vi "Test_PXI_Trig2.vi"() -> ()   [LabVIEW 2018]
uses:
  <vilib>/Platform/TimedLoop/XDataNode/timing_clust.ctl
  <vilib>/Platform/TimedLoop/XDataNode/nitl_modes.ctl
  <vilib>/Platform/TimedLoop/XDataNode/wakeup.ctl
  <vilib>/rvi/Emulation/niFpgaGetClockAttributes.vi
  <vilib>/rvi/Emulation/niFpgaSctlEmulationGetInTimedLoop.vi
  <vilib>/rvi/Emulation/niFpgaEmulationReportErrorSimple.vi
  <vilib>/rvi/eio/common/nirviEmuTemplateMethod_errors.vi
  <vilib>/rvi/Emulation/niFpgaCriticalErrorInLSC.vi
  <vilib>/eio/EIONode/EIONode.xnode
  <vilib>/Platform/TimedLoop/XDataNode/XDataNode.xnode
  <vilib>/Platform/TimedLoop/XDataNode/XDNodeRunTimeDep.lvlib
panel:
  out "PXI_Trig0 read":bool
  in  "PXI_Trig0  write":bool
  in  "Sample Clock Commit":bool
  in  "Sample Clock Select":u8
  out "SPI Idle":bool
  out "Configuration Error":bool
  out "Synthesizer Locked":bool
  out "Configured?":bool
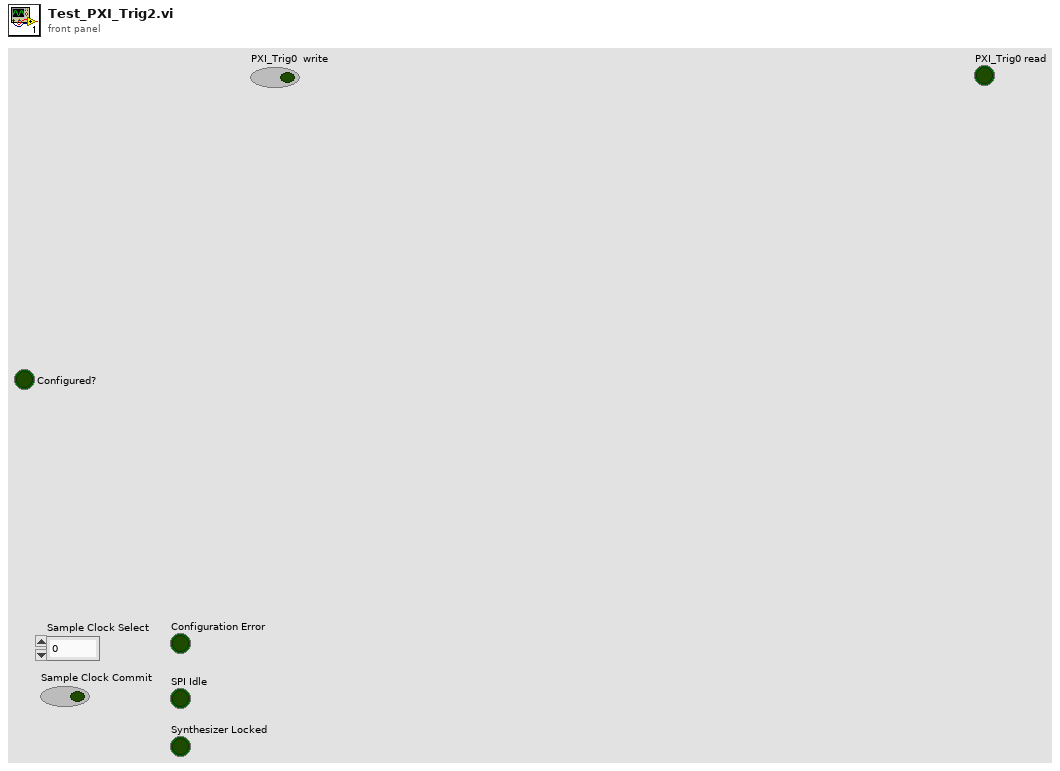
[diagram p1: front panel]
types:
  T1 = typedef "XDNodeRunTimeDep.lvlib/timing_clust.ctl" = cluster{"Expected End [f-1]":u64, "Actual End [f-1]":u64, "Finished Late? [f-1]":bool, "Expected End [i-1]":u64, "Actual End [i-1]":u64, "Finished Late? [i-1]":bool, "Expected Start [i]":u64, "Actual Start [i]":u64, "Expected Start [f]":u64, "Actual Start [f]":u64, "Source Name":string, "Structure Name":string, "Period":i64, "Deadline":i64, "Offset":i64, "Start":i64, "Priority":i32, "Timeout":i32, "Mode":T2, "Wakeup Reason":T3, "Error":errorcluster, "Source Type":string, "Secondary Source Type":string, "Global End Time":u64, "Global Start Time":u64, "Frame Duration":u64, "Iteration Duration":u64, "Assigned CPU":i32, "I/O Scan Engine Mode":u32}
  T2 = typedef "XDNodeRunTimeDep.lvlib/nitl_modes.ctl" = enum32{"No Change", "Process missed periods, maintain original phase", "Discard missed periods, maintain original phase", "Process missed periods, ignore original phase", "Discard missed periods, ignore original phase"}
  T3 = typedef "XDNodeRunTimeDep.lvlib/wakeup.ctl" = enum32{"Normal", "Aborted", "Asynchronous wakeup", "Timing source error", "Timed loop error", "Timeout"}
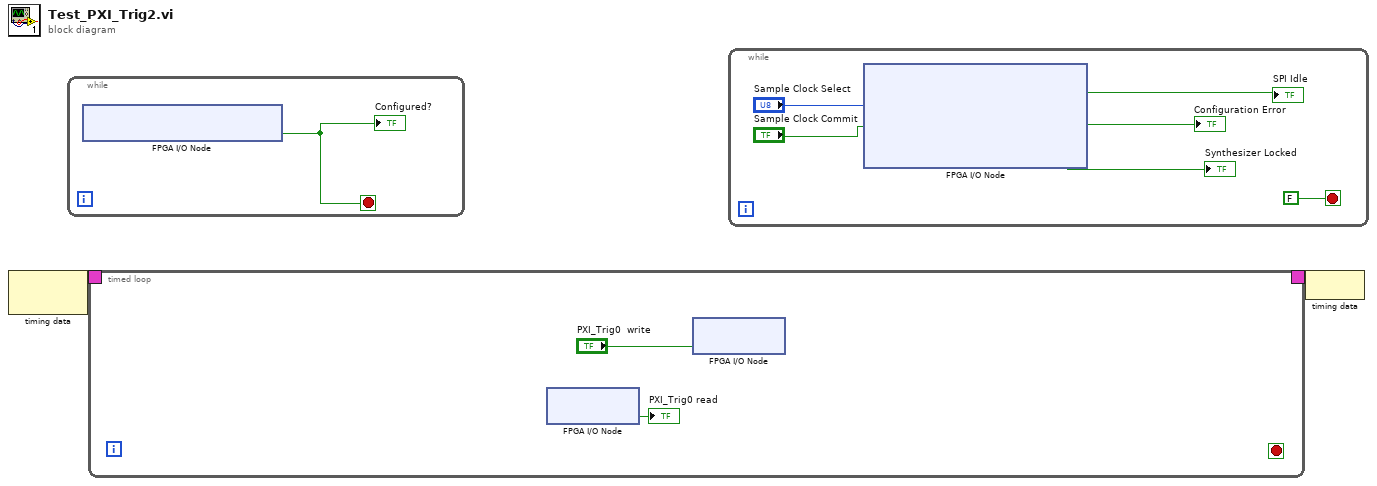
[diagram p0: block diagram]
diagram:
  n1 = node-c288() -> (w2:T1)  [unwired: 1 in]
  n2 = while {
    stop <- w3 stop-if-true
    n3 = xnode "FPGA I/O Node"() -> ("IO Module\\Initialization Done"=w3:bool)  [unwired: 1 in, 1 out]
    "Configured?" <- w3
  }
  n4 = timed-loop {
    timing: w2 -> [_]
    timing-out: [_] -> w1
    stop <- _ stop-if-true
    n5 = xnode "FPGA I/O Node"() -> ("PXI_Trig0"=→"PXI_Trig0 read":bool)  [unwired: 1 in, 1 out]
    n6 = xnode "FPGA I/O Node"("PXI_Trig0"="PXI_Trig0  write") -> ()  [unwired: 1 in, 1 out]
  }
  n7 = while {
    stop <- FALSE stop-if-true
    n8 = xnode "FPGA I/O Node"("IO Module\\Sample Clock Select"="Sample Clock Select", "IO Module\\Sample Clock Commit"="Sample Clock Commit") -> ("IO Module\\SPI Idle"=→"SPI Idle":bool, "IO Module\\Configuration Error"=→"Configuration Error":bool, "IO Module\\Synthesizer Locked"=→"Synthesizer Locked":bool)  [unwired: 5 in, 5 out]
  }
  n9 = node-c288(w1) -> ()
